vi "NCS_IQ_OneTx.vi"(4 "error in":errorcluster, 5 "Coerced IQ rate":dbl, 6 "Waveform Size":dbl, 9 "Channel 0\nTone Frequency":dbl, 10 "Channel 0\nTone Amplitude":dbl) -> (0 "error out":errorcluster, 2 "IQ waveform array":cdb[](array[numeric]), 3 "IQ waveform":waveform(dbl)[](array[waveform]))   [LabVIEW 2016]
uses:
  <vilib>/measure/NI_MABase.lvlib
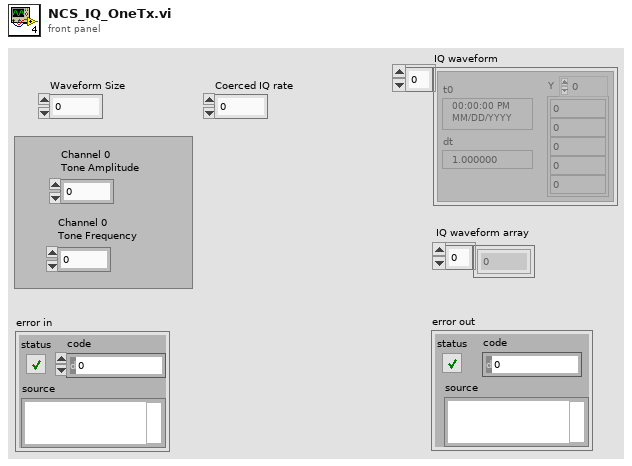
[diagram p1: front panel]
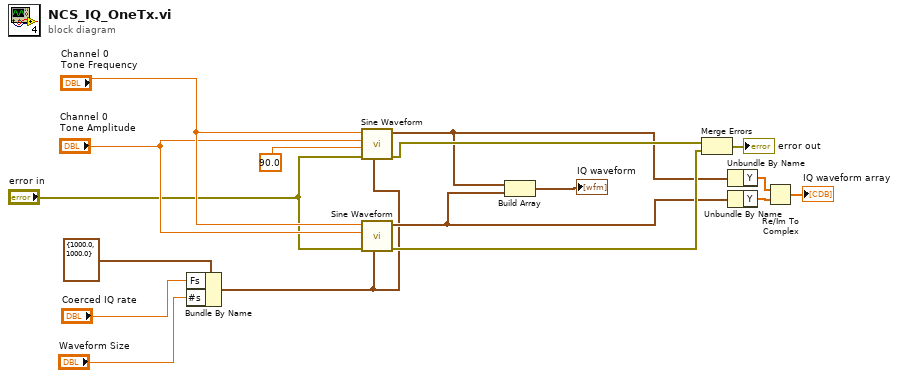
[diagram p0: block diagram]
diagram:
  n1 = Bundle By Name(cluster=cluster{"Fs":dbl, "#s":dbl} {"Fs"=1000.0, "#s"=1000.0} ("sampling info"), "Fs"="Coerced IQ rate", "#s"="Waveform Size") -> (w2:cluster{"Fs":dbl, "#s":dbl})
  n2 = call <vilib>:"Sine Waveform.vi"("sampling info"=w2, "error in (no error)"="error in", "phase"=90.0, "amplitude"="Channel 0\nTone Amplitude", "frequency"="Channel 0\nTone Frequency") -> ("error out"=w14:errorcluster, "signal out"=w5:waveform(dbl))  [unwired: 5 in]
  n3 = call <vilib>:"Sine Waveform.vi"("sampling info"=w2, "error in (no error)"="error in", "amplitude"="Channel 0\nTone Amplitude", "frequency"="Channel 0\nTone Frequency") -> ("error out"=w13:errorcluster, "signal out"=w6:waveform(dbl))  [unwired: 6 in]
  n4 = Build Array(w5, w6) -> (→"IQ waveform":waveform(dbl)[])
  n5 = Merge Errors(w14, w13) -> (→"error out":errorcluster)
  n6 = Unbundle By Name(w5) -> ("Y"=w9:dbl[])
  n7 = Unbundle By Name(w6) -> ("Y"=w10:dbl[])
  n8 = Re/Im To Complex(1:w10, 2:w9) -> (0:→"IQ waveform array":cdb[])
